vi "ExpandExistingGraphAndRedirect.vi"(8 "error in (no error)":errorcluster, 10 "GraphNode in":refnum<data-value>, 11 "Graph in":refnum<class "Graph.lvclass">) -> (0 "error out":errorcluster, 1 "ExpandedNodes":refnum<data-value>[](array[refnum]), 2 "GraphNode out":refnum<data-value>, 3 "Graph out":refnum<class "Graph.lvclass">)   [LabVIEW 2009, in "Graph.lvclass"]
uses:
  Graph.lvclass
  GraphNode/GraphNode.lvclass
  LinkedList/LinkedList.lvclass
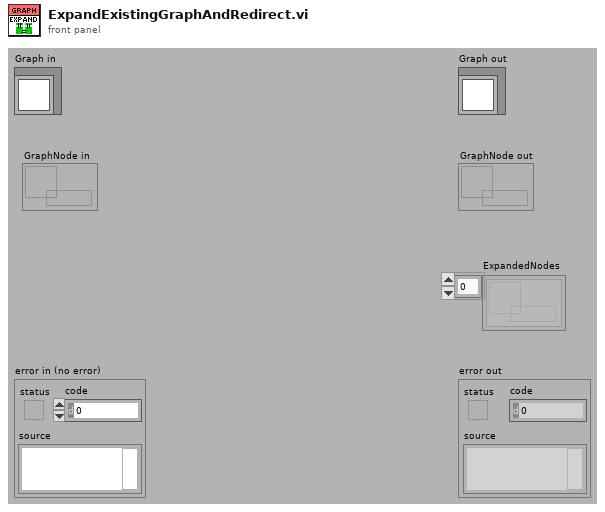
[diagram p1: front panel]
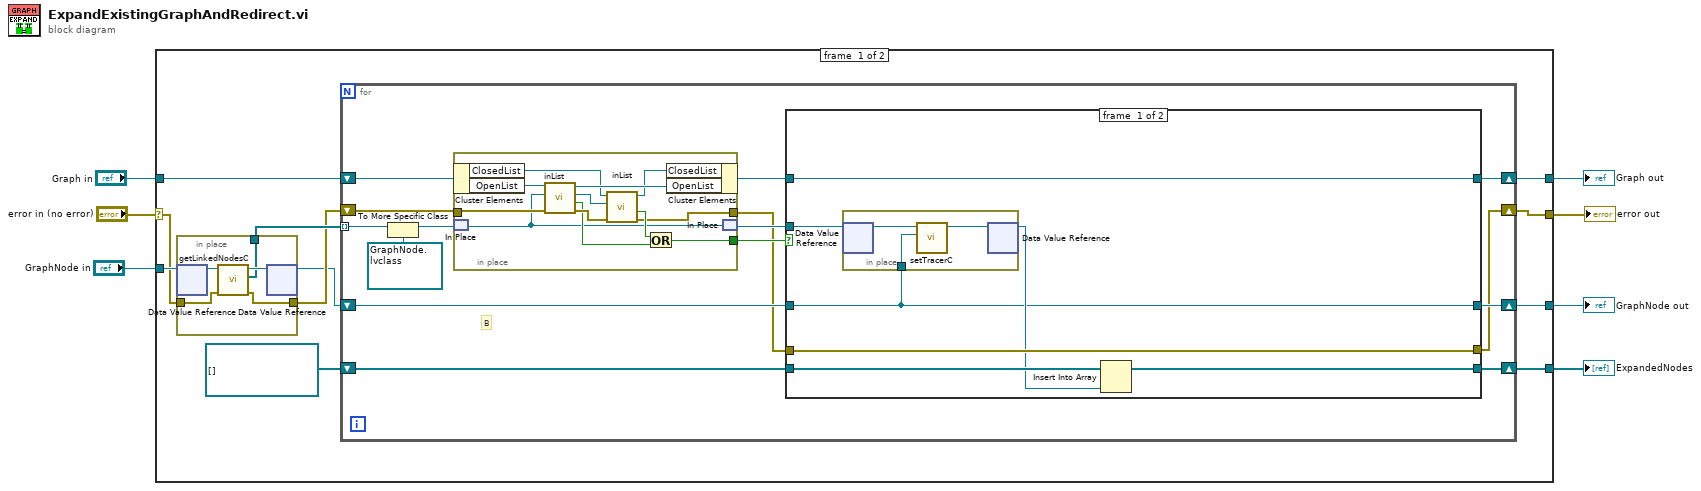
[diagram p0: block diagram]
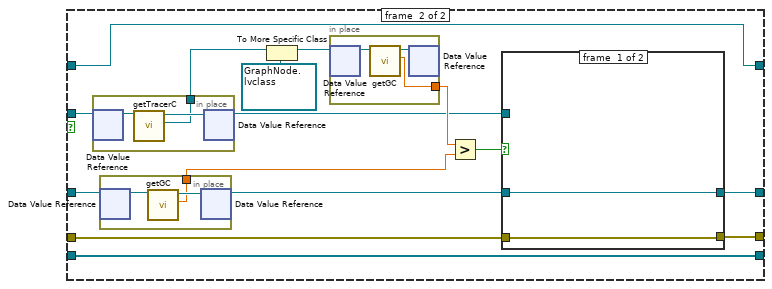
[diagram p2: hidden frame]
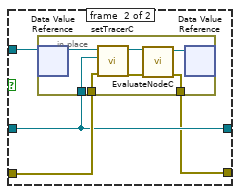
[diagram p3: hidden frame]
diagram:
  n1 = case shown="No Error" "error in (no error)" {
    selector: "error in (no error)" -> [w17 w100]
    tunnel: [w8 w100] -> w6
    tunnel: [w11 w99] -> w4
    tunnel: "Graph in" -> [w15 w99]
    tunnel: "GraphNode in" -> [w18 w98]
    tunnel: [w10 _] -> w2
    tunnel: [w9 w98] -> w1
    frame #0 {
      n2 = in-place {
        in-place-border: w17 -> [w96]
        in-place-border: [w95] -> w14
        in-place-border: [w93] -> w16
        n3 = in-place-dvr #1(w18) -> (w97:refnum<class "GraphNode.lvclass">)  [unwired: 1 out]
        n4 = call "getLinkedNodesC.vi"("error in (no error)"=w96, "GraphNode in"=w97) -> ("error out"=w95:errorcluster, "LinkedNodes"=w93:refnum<data-value>[], "GraphNode out"=w94:refnum<class "GraphNode.lvclass">)  [unwired: 7 in]
        n5 = in-place-dvr #1(w94) -> (w12:refnum<data-value>)  [unwired: 1 out]
      }
      n6 = for {
        tunnel: w16 -> [w31] mode=indexing
        shift-right: [w23] -> w11
        shift-left: w15 -> [w32]
        shift-right: [w24] -> w10
        shift-left: refnum<data-value>[] [] -> [w25]
        shift-right: [w20] -> w9
        shift-left: w12 -> [w22]
        shift-right: [w19] -> w8
        shift-left: w14 -> [w30]
        # "B"
        n7 = To More Specific Class(target class=refnum<data-value> refnum ("GraphNode out 2"), reference=w31) -> (specific class reference=w29:refnum<data-value>)  [unwired: 1 in, 1 out]
        n8 = in-place {
          in-place-border: w30 -> [w90]
          in-place-border: [w82] -> w28
          in-place-border: [w81] -> w21
          n9 = in-place-cluster #2(w32) -> ("ClosedList"=w89:refnum<class "BasicSortedList.lvclass">, "OpenList"=w92:refnum<class "BasicSortedList.lvclass">)
          n10 = in-place-match #3(w29) -> (w83:refnum<data-value>)
          n11 = call "inList.vi"("error in (no error)"=w90, "LLNode in"=w83, "LinkedList in"=w92) -> ("error out"=w86:errorcluster, "inList"=w84:bool, "LLNode out"=w87:refnum<data-value>, "LinkedList out"=w91:refnum<class "BasicSortedList.lvclass">)  [unwired: 4 in, 1 out]
          n12 = call "inList.vi"("error in (no error)"=w86, "LLNode in"=w87, "LinkedList in"=w89) -> ("error out"=w81:errorcluster, "inList"=w85:bool, "LinkedList out"=w88:refnum<class "BasicSortedList.lvclass">)  [unwired: 4 in, 2 out]
          n13 = Or(x=w85, y=w84) -> (x .or. y?=w82:bool)
          n14 = in-place-cluster #2("ClosedList"=w88, "OpenList"=w91) -> (w27:refnum<class "Graph.lvclass">)
          n15 = in-place-match #3(w83) -> (w26:refnum<data-value>)
        }
        n16 = case shown="True" w28 {
          tunnel: w27 -> [w38 w52]
          tunnel: w26 -> [w36 w56]
          tunnel: w25 -> [w40 w58]
          tunnel: [w39 w58] -> w24
          tunnel: [w38 w52] -> w23
          tunnel: w22 -> [w34 w57]
          tunnel: w21 -> [w37 w46]
          tunnel: [w34 w45] -> w20
          tunnel: [w37 w44] -> w19
          frame #0 {
            n17 = in-place {
              in-place-border: w34 -> [w41]
              n18 = in-place-dvr #4(w36) -> (w43:refnum<class "GraphNode.lvclass">)  [unwired: 1 out]
              n19 = call "setTracerC.vi"("tracer"=w41, "GraphNode in"=w43) -> ("GraphNode out"=w42:refnum<class "GraphNode.lvclass">)  [unwired: 8 in, 1 out]
              n20 = in-place-dvr #4(w42) -> (w35:refnum<data-value>)  [unwired: 1 out]
            }
            n21 = Insert Into Array(array=w40, new element=w35) -> (w39:refnum<data-value>[])  [unwired: 1 in]
          }
          frame #1 {
            n22 = in-place {
              in-place-border: [w75] -> w55
              n23 = in-place-dvr #5(w56) -> (w77:refnum<class "GraphNode.lvclass">)  [unwired: 1 out]
              n24 = call "getTracerC.vi"("GraphNode in"=w77) -> ("tracer"=w75:refnum<data-value>, "GraphNode out"=w76:refnum<class "GraphNode.lvclass">)  [unwired: 8 in, 1 out]
              n25 = in-place-dvr #5(w76) -> (w48:refnum<data-value>)  [unwired: 1 out]
            }
            n26 = in-place {
              in-place-border: [w78] -> w50
              n27 = in-place-dvr #6(w57) -> (w80:refnum<class "GraphNode.lvclass">)  [unwired: 1 out]
              n28 = call "getGC.vi"("GraphNode in"=w80) -> ("G"=w78:dbl, "GraphNode out"=w79:refnum<class "GraphNode.lvclass">)  [unwired: 8 in, 1 out]
              n29 = in-place-dvr #6(w79) -> (w47:refnum<data-value>)  [unwired: 1 out]
            }
            n30 = To More Specific Class(target class=refnum<data-value> refnum ("GraphNode out 2"), reference=w55) -> (specific class reference=w53:refnum<data-value>)  [unwired: 1 in, 1 out]
            n31 = in-place {
              in-place-border: [w74] -> w51
              n32 = in-place-dvr #7(w53) -> (w72:refnum<class "GraphNode.lvclass">)  [unwired: 1 out]
              n33 = call "getGC.vi"("GraphNode in"=w72) -> ("G"=w74:dbl, "GraphNode out"=w73:refnum<class "GraphNode.lvclass">)  [unwired: 8 in, 1 out]
              n34 = in-place-dvr #7(w73) -> ()  [unwired: 2 out]
            }
            n35 = Greater?(x=w51, y=w50) -> (0:w49:bool)
            n36 = case shown="True" w49 {
              tunnel: w48 -> [_ w64]
              tunnel: w47 -> [w60 w62]
              tunnel: w46 -> [w59 w63]
              tunnel: [w60 w62] -> w45
              tunnel: [w59 w61] -> w44
              frame #0 {
              }
              frame #1 {
                n37 = in-place {
                  in-place-border: w62 -> [w70]
                  in-place-border: w63 -> [w66]
                  in-place-border: [w65] -> w61
                  n38 = in-place-dvr #8(w64) -> (w71:refnum<class "GraphNode.lvclass">)  [unwired: 1 out]
                  n39 = call "setTracerC.vi"("error in (no error)"=w66, "tracer"=w70, "GraphNode in"=w71) -> ("error out"=w67:errorcluster, "GraphNode out"=w69:refnum<class "GraphNode.lvclass">)  [unwired: 7 in]
                  n40 = call "EvaluateNodeC.vi"("error in (no error)"=w67, "GraphNode in"=w69) -> ("error out"=w65:errorcluster, "GraphNode out"=w68:refnum<class "GraphNode.lvclass">)  [unwired: 8 in]
                  n41 = in-place-dvr #8(w68) -> ()  [unwired: 2 out]
                }
              }
            }
          }
        }
      }
    }
    frame #1 {
    }
  }
  "error out" <- w6
  "Graph out" <- w4
  "GraphNode out" <- w1
  "ExpandedNodes" <- w2
